vi "Agilent VNA Read Status Bytes.vi"(7 "Agilent VNA":T1, 8 "error in (no error)":errorcluster, 10 "STB Only? (f: Read registers)":bool, 11 "VISA Resource Name":refnum<visa-resource-name>) -> (0 "error out":errorcluster, 1 "Event Status Register B":bool[](array[boolean]), 2 "Event Status Register":bool[](array[boolean]), 3 "dup VISA Resource Name":refnum<visa-resource-name>, 4 "Status Byte":bool[](array[boolean]))   [LabVIEW 2011]
doc: "This VI for the HP8753B Network Analyzer reads the status byte and the two event status registers. The two status registers are read out as regular output and will therefore clear anything already in the output queue."
uses:
  TypeDefs/Agilent VNA Instrument Info.ctl
panel:
  # "read status byte only\nread status byte and status registers"
  # "Single, Num of Groups, or Cal Standard Complete\n\nService Routine Waiting\n\nData Entry Complete\n\nLimit Failed CH 2\n\nLimit Failed CH 1\n\nSearch Fail CH 2\n\nSearch Fail CH 1\n\nALC Unlock"
  # "Operation Complete\n\nRequest Control\n\nQuery Error\n\n\n\nExecution Error\n\nSyntax Error (GP-IB)\n\nUser Request\n\nPower On"
  # "Reverse GET\n\nForward GET\n\nEvent Status Register B\n\nCheck Error Queue\n\nMessage in Output Queue\n\nEvent Status Register\n\nRequest Service"
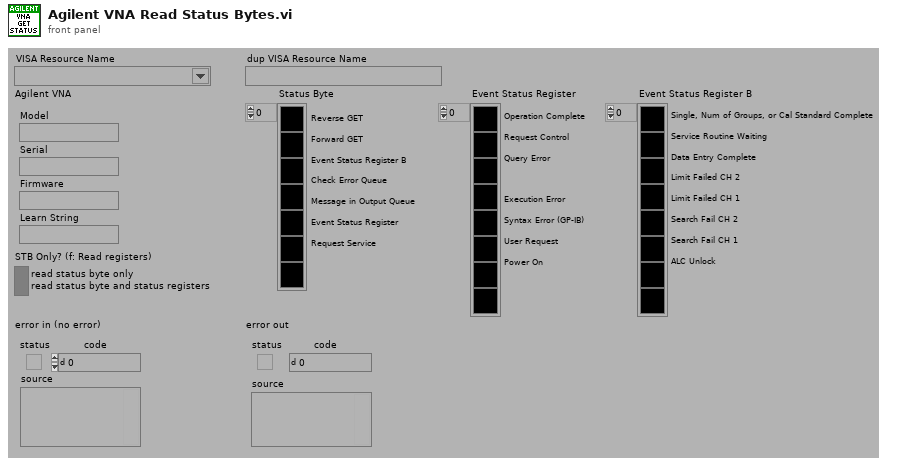
[diagram p1: front panel]
types:
  T1 = typedef "Agilent VNA Instrument Info.ctl" = cluster{"Model":string, "Serial":string, "Firmware":string, "Learn String":string}
  T2 = typedef "Agilent VNA Model.ctl" = enum16{"Not Supported", "8510X", "8719X", "8720X", "8722X", "8753X", "ENA", "PNA", "Field Fox"}
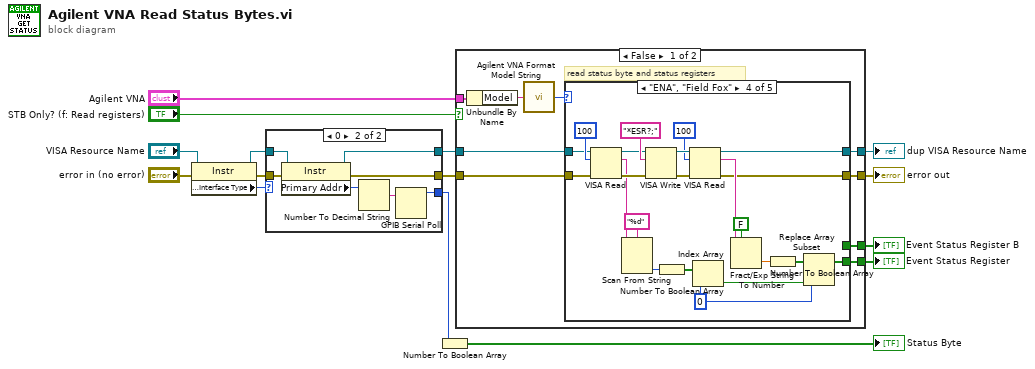
[diagram p0: block diagram]
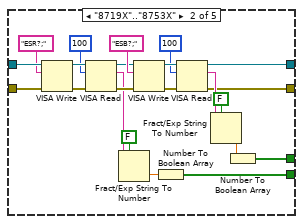
[diagram p4: hidden frame]
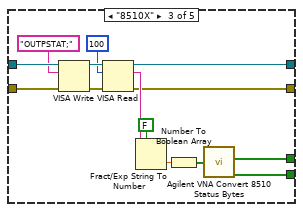
[diagram p5: hidden frame]
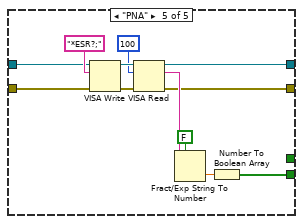
[diagram p6: hidden frame]
diagram:
  n1 = property class="Instr"(reference="VISA Resource Name", error in="error in (no error)") -> (reference out=w4:refnum<visa-resource-name>, error out=w2:errorcluster, "Interface Information:Interface Type"=w1:u16)
  n2 = case shown="0" w1 {
    tunnel: [_ w24] -> w14
    tunnel: w4 -> [w17 w21]
    tunnel: [w17 w20] -> w13
    tunnel: [w16 w19] -> w10
    tunnel: w2 -> [w16 w18]
    frame Default {
    }
    frame 0 {
      n3 = property class="Instr"(reference=w21, error in=w18) -> (reference out=w20:refnum<visa-resource-name>, error out=w19:errorcluster, "Primary Addr"=w22:u16)
      n4 = Number To Decimal String(number=w22) -> (decimal integer string=w23:string)  [unwired: 1 out]
      n5 = GPIB Serial Poll(0:w23) -> (2:w24:i16)  [unwired: 1 in, 2 out]
    }
  }
  n6 = Number To Boolean Array(number=w14) -> (Boolean array=→"Status Byte":bool[])
  n7 = case shown="False" "STB Only? (f: Read registers)" {
    tunnel: w13 -> [w32 w107]
    tunnel: w10 -> [w33 w106]
    tunnel: [w31 w107] -> w12
    tunnel: [w30 w106] -> w11
    tunnel: "Agilent VNA" -> [w26 _]
    tunnel: [w28 _] -> w7
    tunnel: [w27 _] -> w6
    frame False {
      # "read status byte and status registers"
      n8 = Unbundle By Name(w26) -> ("Model"=w25:string)
      n9 = call "Agilent VNA Format Model String.vi"("Model"=w25) -> ("Model"=w29:T2)
      n10 = case shown="\"ENA\", \"Field Fox\"" w29 {
        tunnel: w33 -> [w34 w57 w71 w81 w95]
        tunnel: w32 -> [w35 w56 w70 w83 w94]
        tunnel: [_ w55 w59 _ _] -> w28
        tunnel: [_ w54 w58 w77 w96] -> w27
        tunnel: [w35 w43 w61 w85 w97] -> w31
        tunnel: [w34 w42 w62 w86 w98] -> w30
        frame "Not Supported" {
        }
        frame "8719X".."8753X" {
          n11 = VISA Write(VISA resource name=w56, write buffer="ESR?;", error in (no error)=w57) -> (VISA resource name out=w39:refnum<visa-resource-name>, error out=w46:errorcluster)  [unwired: 1 out]
          n12 = VISA Read(VISA resource name=w39, byte count=u32 100, error in (no error)=w46) -> (VISA resource name out=w51:refnum<visa-resource-name>, read buffer=w44:string, error out=w52:errorcluster)  [unwired: 1 out]
          n13 = Fract/Exp String To Number(use system decimal point (T)=FALSE, string=w44) -> (number=w45:dbl)  [unwired: 3 out]
          n14 = VISA Write(VISA resource name=w51, write buffer="ESB?;", error in (no error)=w52) -> (VISA resource name out=w41:refnum<visa-resource-name>, error out=w48:errorcluster)  [unwired: 1 out]
          n15 = Number To Boolean Array(number=w45) -> (Boolean array=w54:bool[])
          n16 = VISA Read(VISA resource name=w41, byte count=u32 100, error in (no error)=w48) -> (VISA resource name out=w43:refnum<visa-resource-name>, read buffer=w50:string, error out=w42:errorcluster)  [unwired: 1 out]
          n17 = Fract/Exp String To Number(use system decimal point (T)=FALSE, string=w50) -> (number=w49:dbl)  [unwired: 3 out]
          n18 = Number To Boolean Array(number=w49) -> (Boolean array=w55:bool[])
        }
        frame "8510X" {
          n19 = VISA Write(VISA resource name=w70, write buffer="OUTPSTAT;", error in (no error)=w71) -> (VISA resource name out=w65:refnum<visa-resource-name>, error out=w68:errorcluster)  [unwired: 1 out]
          n20 = VISA Read(VISA resource name=w65, byte count=u32 100, error in (no error)=w68) -> (VISA resource name out=w61:refnum<visa-resource-name>, read buffer=w66:string, error out=w62:errorcluster)  [unwired: 1 out]
          n21 = Fract/Exp String To Number(use system decimal point (T)=FALSE, string=w66) -> (number=w67:dbl)  [unwired: 3 out]
          n22 = Number To Boolean Array(number=w67) -> (Boolean array=w60:bool[])
          n23 = call "Agilent VNA Convert 8510 Status Bytes.vi"("8510 Status Bytes"=w60) -> ("Event Status Register B"=w59:bool[], "Event Status Register"=w58:bool[])  [unwired: 6 out]
        }
        frame "ENA", "Field Fox" {
          w72 = 0 ("index")
          n24 = VISA Read(VISA resource name=w83, byte count=u32 100, error in (no error)=w81) -> (VISA resource name out=w82:refnum<visa-resource-name>, read buffer=w75:string, error out=w80:errorcluster)  [unwired: 1 out]
          n25 = Scan From String(format string="%d", input string=w75) -> (output 1=w76:i32)  [unwired: 2 in, 4 out]
          n26 = VISA Write(VISA resource name=w82, write buffer="*ESR?;", error in (no error)=w80) -> (VISA resource name out=w89:refnum<visa-resource-name>, error out=w92:errorcluster)  [unwired: 1 out]
          n27 = Number To Boolean Array(number=w76) -> (Boolean array=w74:bool[])
          n28 = VISA Read(VISA resource name=w89, byte count=u32 100, error in (no error)=w92) -> (VISA resource name out=w85:refnum<visa-resource-name>, read buffer=w90:string, error out=w86:errorcluster)  [unwired: 1 out]
          n29 = Index Array(array=w74, index=w72) -> (element=w73:bool)
          n30 = Fract/Exp String To Number(use system decimal point (T)=FALSE, string=w90) -> (number=w91:dbl)  [unwired: 3 out]
          n31 = Number To Boolean Array(number=w91) -> (Boolean array=w78:bool[])
          n32 = Replace Array Subset(array=w78, new element=w73, index=w72) -> (w77:bool[])
        }
        frame "PNA" {
          n33 = VISA Write(VISA resource name=w94, write buffer="*ESR?;", error in (no error)=w95) -> (VISA resource name out=w101:refnum<visa-resource-name>, error out=w104:errorcluster)  [unwired: 1 out]
          n34 = VISA Read(VISA resource name=w101, byte count=u32 100, error in (no error)=w104) -> (VISA resource name out=w97:refnum<visa-resource-name>, read buffer=w102:string, error out=w98:errorcluster)  [unwired: 1 out]
          n35 = Fract/Exp String To Number(use system decimal point (T)=FALSE, string=w102) -> (number=w103:dbl)  [unwired: 3 out]
          n36 = Number To Boolean Array(number=w103) -> (Boolean array=w96:bool[])
        }
      }
    }
    frame True {
      # "read status byte only"
    }
  }
  "dup VISA Resource Name" <- w12
  "error out" <- w11
  "Event Status Register B" <- w7
  "Event Status Register" <- w6
